vi "FP_Size Inside Bounds with Scrollbars.vi"(7 "WkSpace":T1, 8 "Error":errorcluster, 11 "VI":refnum<vi>) -> (0 "Error Out":errorcluster, 2 "Fit Successful":bool, 3 "VI Out":refnum<vi>)   [LabVIEW 2020]
uses:
  <vilib>/Utility/miscctls.llb/LVRectTypeDef.ctl
  TypeDefs_Utility/Cluster_FP_Scroll Bars Hide Show.ctl
  TypeDefs_Utility/ENUM_FP_Show-Hide Select.ctl
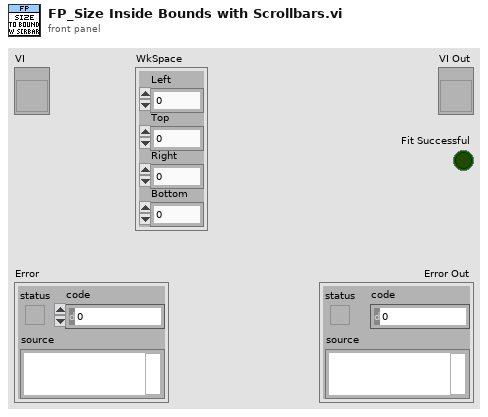
[diagram p1: front panel]
types:
  T1 = typedef "LVRectTypeDef.ctl" = cluster{"Left":i16, "Top":i16, "Right":i16, "Bottom":i16}
  T2 = typedef "Cluster_FP_Scroll Bars Hide Show.ctl" = cluster{"Horiz SBar":T3, "Vert SBar":T3}
  T3 = typedef "ENUM_FP_Show-Hide Select.ctl" = enum16{"No Change", "Hide", "Show"}
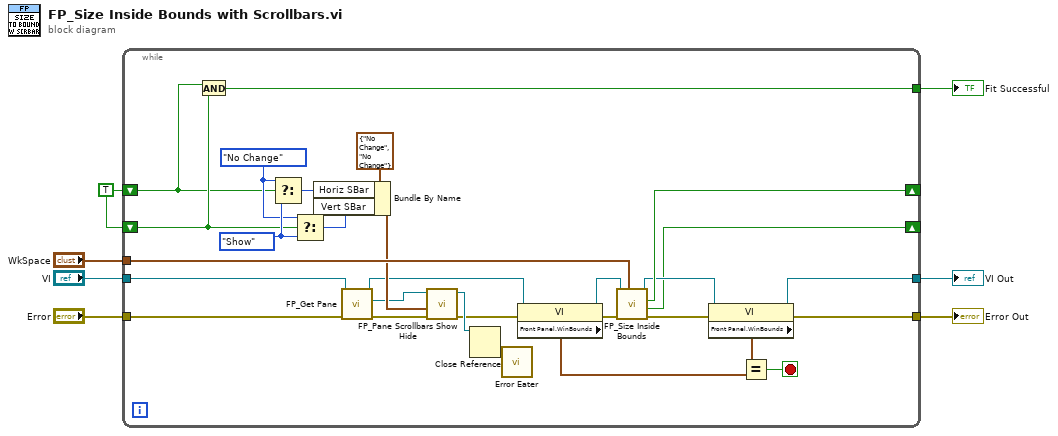
[diagram p0: block diagram]
diagram:
  w1 = TRUE ("Horizontal In Range Out")
  n1 = while {
    tunnel: [w12] -> w7
    tunnel: "VI" -> [w21]
    tunnel: "Error" -> [w20]
    tunnel: [w14] -> w4
    tunnel: [w36] -> w3
    tunnel: "WkSpace" -> [w35]
    shift-right: [w34] -> _
    shift-left: w1 -> [w22]
    shift-right: [w11] -> _
    shift-left: w1 -> [w23]
    stop <- w8 stop-if-true
    w25 = ENUM_FP_Show-Hide_Select."Show" ("Horizontal")
    w24 = ENUM_FP_Show-Hide_Select."No Change" ("Horizontal")
    n2 = And(x=w22, y=w23) -> (x .and. y?=w36:bool)
    n3 = Select(t=w24, s=w22, f=w25) -> (s? t:f=w30:T3)
    n4 = Select(t=w24, s=w23, f=w25) -> (s? t:f=w29:T3)
    n5 = Bundle By Name(cluster=T2 {"Horiz SBar"=enum."No Change", "Vert SBar"=enum."No Change"} ("Scrollbar Settings"), "Horiz SBar"=w30, "Vert SBar"=w29) -> (w31:T2)
    n6 = call "FP_Get Pane.vi"("Error"=w20, "VI"=w21) -> ("Error Out"=w26:errorcluster, "Pane Refnum Out"=w28:refnum<vi>, "VI Out"=w19:refnum<vi>)  [unwired: 7 in]
    n7 = call "FP_Pane Scrollbars Show Hide.vi"("Error"=w26, "Scrollbar Settings"=w31, "Pane"=w28) -> ("Error Out"=w17:errorcluster, "Pane Out"=w27:refnum<vi>)  [unwired: 7 in]
    n8 = Close Reference(reference=w27) -> (error out=w33:errorcluster)  [unwired: 1 in]
    n9 = call "Error Eater.vi"("error in (no error)"=w33) -> ()  [unwired: 2 in]
    n10 = property class="VI"(reference=w19, error in=w17) -> (reference out=w18:refnum<vi>, error out=w16:errorcluster, "Front Panel.WinBounds"=w9:T1)
    n11 = call "FP_Size Inside Bounds.vi"("Work Space"=w35, "Error"=w16, "VI Ref"=w18) -> ("Error Out"=w15:errorcluster, "Vertical In Range Out"=w11:bool, "Horizontal In Range Out"=w34:bool, "VI Ref Out"=w13:refnum<vi>)  [unwired: 3 in, 2 out]
    n12 = property class="VI"(reference=w13, error in=w15) -> (reference out=w12:refnum<vi>, error out=w14:errorcluster, "Front Panel.WinBounds"=w10:T1)
    n13 = Equal?(x=w10, y=w9) -> (x = y?=w8:bool)
  }
  "VI Out" <- w7
  "Fit Successful" <- w3
  "Error Out" <- w4
